vi "Intersect Rectangle.vi"(1 "Rectangle B":T1, 2 "Rectangle A":T1) -> (0 "Intersect Rectangle":T1)   [LabVIEW 2020, in "Map Model.lvlib" / "Tool.lvclass"]
uses:
  Tool.lvclass
panel:
  # "NOTICE -- YOU MUST LEAVE THIS NOTICE IN PLACE.\n\nCopyright (c) 2017, LIANG LIU Shawn.Liu.cn@gmail.com\nAll rights reserved.\n\nRedistribution and use in source and binary forms, with or without modification, are permitted provided that the following conditions are met:\n-Redistributions of source code must retain the above copyright notice, this list of conditions and the following disclaimer.\n-Redistributions in binary form must reproduce the above copyright notice, this list of conditions and the following disclaimer in the documentation and/or other materials provided with the distribution.\n-Neither the name of the eLp nor the names of its contributors may be used to endorse or promote products derived from this software without specific prior written permission.\n\nTHIS SOFTWARE IS PROVIDED BY THE COPYRIGHT HOLDERS AND CONTRIBUTORS \"AS IS\" AND ANY EXPRESS OR IMPLIED WARRANTIES, INCLUDING, BUT NOT LIMITED TO, THE IMPLIED WARRANTIES OF MERCHANTABILITY AND FITNESS FOR A PARTICULAR PURPOSE ARE DISCLAIMED. IN NO EVENT SHALL THE COPYRIGHT HOLDER OR CONTRIBUTORS BE LIABLE FOR ANY DIRECT, INDIRECT, INCIDENTAL, SPECIAL, EXEMPLARY, OR CONSEQUENTIAL DAMAGES (INCLUDING, BUT NOT LIMITED TO, PROCUREMENT OF SUBSTITUTE GOODS OR SERVICES; LOSS OF USE, DATA, OR PROFITS; OR BUSINESS INTERRUPTION) HOWEVER CAUSED AND ON ANY THEORY OF LIABILITY, WHETHER IN CONTRACT, STRICT LIABILITY, OR TORT (INCLUDING NEGLIGENCE OR OTHERWISE) ARISING IN ANY WAY OUT OF THE USE OF THIS SOFTWARE, EVEN IF ADVISED OF THE POSSIBILITY OF SUCH DAMAGE."
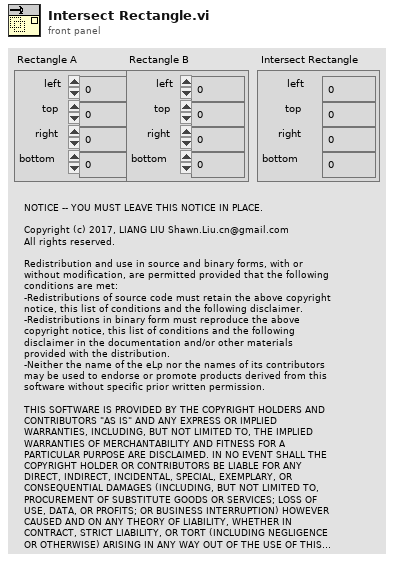
[diagram p1: front panel]
types:
  T1 = cluster{"left":i16, "top":i16, "right":i16, "bottom":i16}
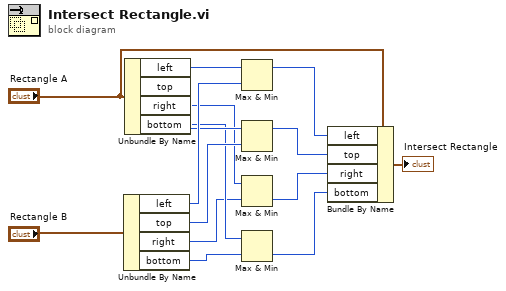
[diagram p0: block diagram]
diagram:
  n1 = Unbundle By Name("Rectangle B") -> ("left"=w11:i16, "top"=w9:i16, "right"=w5:i16, "bottom"=w6:i16)
  n2 = Unbundle By Name("Rectangle A") -> ("left"=w12:i16, "top"=w10:i16, "right"=w8:i16, "bottom"=w7:i16)
  n3 = Max & Min(x=w12, y=w11) -> (max(x,y)=w4:i16)  [unwired: 1 out]
  n4 = Max & Min(x=w10, y=w9) -> (max(x,y)=w3:i16)  [unwired: 1 out]
  n5 = Max & Min(x=w8, y=w5) -> (min(x,y)=w2:i16)  [unwired: 1 out]
  n6 = Max & Min(x=w7, y=w6) -> (min(x,y)=w1:i16)  [unwired: 1 out]
  n7 = Bundle By Name(cluster="Rectangle A", "left"=w4, "top"=w3, "right"=w2, "bottom"=w1) -> (→"Intersect Rectangle":T1)
